vi "LV to ITX  Retrieve - HY TDMS.vi"(0 "File or Folder Path":path=path "C:/", 1 "Data Type":T2=enum."DAT", 2 "DAT header length":i32=11, 5 "offset":i32, 7 "length":i32=1, 9 "index":T3={"A"=1, "B"=0, "C"=2, "D"=0, "E"=3, "N1"=0, "N2"=0, "N3"=0, "N4"=0}, 11 "error in (no error)":errorcluster) -> (4 "A vs B":cluster{dbl[], dbl[]}[](graph), 6 "C vs D":cluster{dbl[], dbl[]}[](graph), 8 "E":dbl[][](graph), 10 "N":cluster{"N1":dbl, "N2":dbl, "N3":dbl, "N4":dbl}={"N1"=0.0624995231628418, "N2"=0.0624995231628418, "N3"=0.0624995231628418, "N4"=0.0624995231628418} {"N4" format="%#_6p"; "N3" format="%#_6p"; "N2" format="%#_6p"; "N1" format="%#_6p"}, 14 "Comments":string)   [LabVIEW 2016]
uses:
  <vilib>/Utility/miscctls.llb/LVOffsetAndMultiplierTypeDef.ctl
  <userlib>/LevyLab/LV to ITX/Typedefs/Retrieve Data Type.ctl
  <userlib>/LevyLab/LV to ITX/LVtoITX.lvclass
  <userlib>/LevyLab/Graph Utilities/graph_utilities.lvclass
panel:
  out "First element":dbl
  in  "X min & max":cluster{"Min":dbl, "Max":dbl}
  out "size(s)":i32[](array[numeric])
  out "last element":dbl
  in  "Manual input offset & multiplier for Ex ?":bool
  out "X Scale.Offset and Multiplier":T1
  in  "Specify data section ?":bool
  in  "Data length":i32=5000
  in  "Data offset":i32
  in  "D  is time?":bool
  in  "B is time?":bool
  out "time":string[][](table)
  in  "Use Folder Index File?":bool
  in  "Generate Folder Index File?":bool
  in  "Ez name":string="Ez name"
  in  "Ey name":string="Ey name"
  in  "Ex name":string="Ex name"
  in  "C y name":string="C y name"
  in  "D x name":string="D x name"
  in  "A y name":string="A y name"
  in  "B x name":string="B x name"
  out "Index, Wavenames":string[][](table)
  in  "recolor traces?":bool
  in  "Ex":T1={"Offset"=0.0, "Multiplier"=1.0}
  in  "Ey":T1={"Offset"=0.0, "Multiplier"=1.0}
  out "Path":path
  out "counter":i32
  out "pattern":string="*.dat"
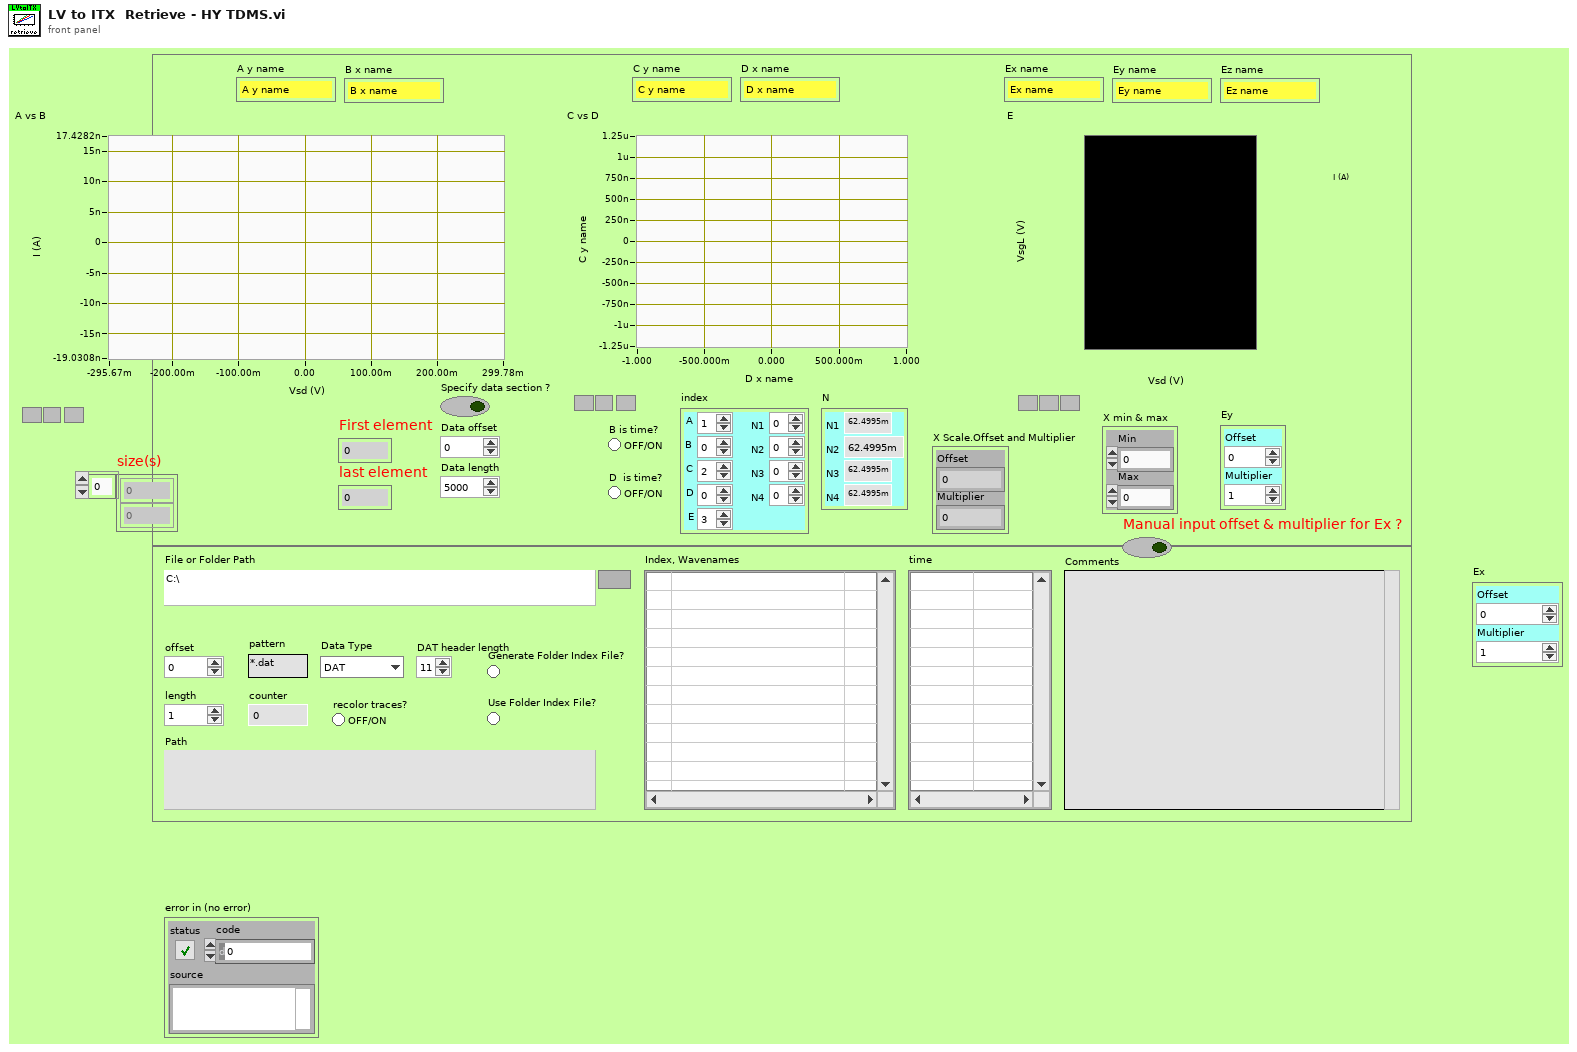
[diagram p1: front panel]
types:
  T1 = typedef "LVOffsetAndMultiplierTypeDef.ctl" = cluster{"Offset":dbl, "Multiplier":dbl}
  T2 = typedef "LVtoITX.lvclass/Retrieve Data Type.ctl" = enum16{"ITX", "ITX w/ 2D", "DAT", "TDMS"}
  T3 = cluster{"A":i32, "B":i32, "C":i32, "D":i32, "E":i32, "N1":i32, "N2":i32, "N3":i32, "N4":i32}
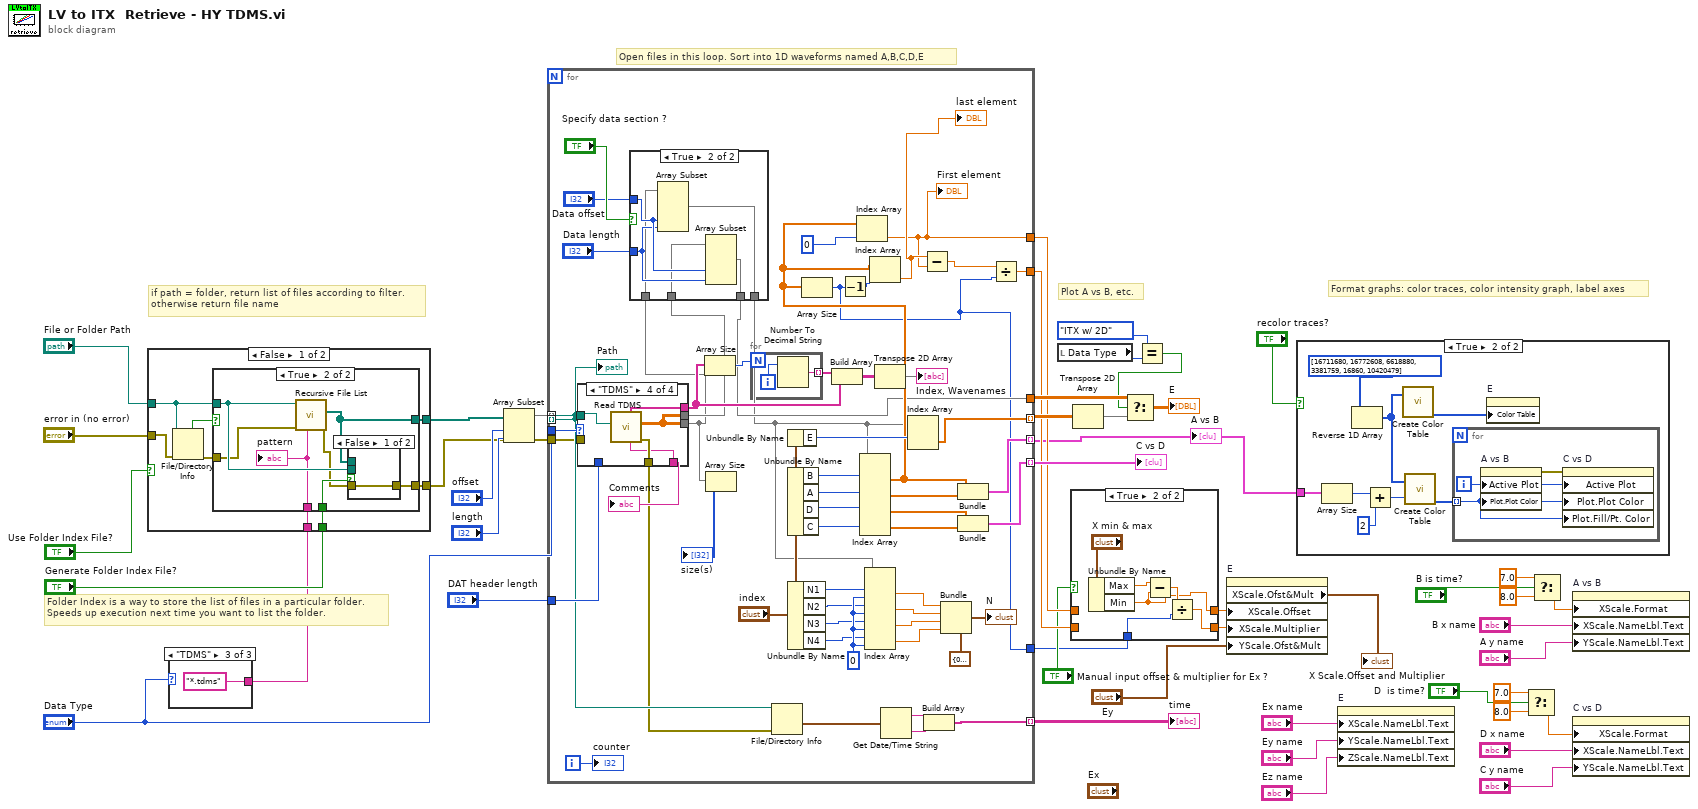
[diagram p0: block diagram]
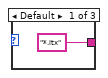
[diagram p3: hidden frame]
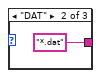
[diagram p4: hidden frame]
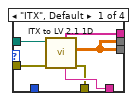
[diagram p7: hidden frame]
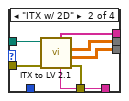
[diagram p8: hidden frame]
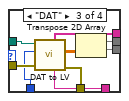
[diagram p9: hidden frame]
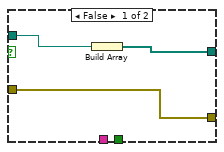
[diagram p10: hidden frame]
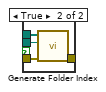
[diagram p11: hidden frame]
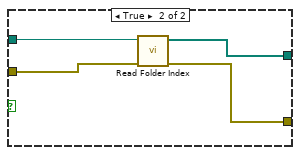
[diagram p12: hidden frame]
diagram:
  # "Plot A vs B, etc."
  # "Format graphs: color traces, color intensity graph, label axes"
  # "Open files in this loop. Sort into 1D waveforms named A,B,C,D,E"
  # "Folder Index is a way to store the list of files in a particular folder.\nSpeeds up execution next time you want to list the folder."
  # "if path = folder, return list of files according to filter.\notherwise return file name"
  n1 = case shown="\"TDMS\"" "Data Type" {
    tunnel: ["*.itx" ("pattern") "*.dat" ("pattern") "*.tdms" ("pattern")] -> w12
    frame Default {
    }
    frame "DAT" {
    }
    frame "TDMS" {
    }
  }
  n2 = case shown="False" "Use Folder Index File?" {
    tunnel: [w55 w75] -> w44
    tunnel: "File or Folder Path" -> [w57 w76]
    tunnel: "Generate Folder Index File?" -> [w54 _]
    tunnel: w12 -> [w53 _]
    tunnel: "error in (no error)" -> [w52 w74]
    tunnel: [w50 w73] -> w9
    frame False {
      n3 = File/Directory Info(path=w57, error in=w52) -> (directory=w56:bool, error out=w51:errorcluster)  [unwired: 5 out]
      n4 = case shown="True" w56 {
        tunnel: [w60 w66] -> w55
        tunnel: w57 -> [w59 w67]
        tunnel: w54 -> [_ w63]
        tunnel: w53 -> [_ w65]
        tunnel: w51 -> [w58 w64]
        tunnel: [w58 w61] -> w50
        frame False {
          n5 = Build Array(w59) -> (w60:path[])
        }
        frame True {
          n6 = call <vilib>:"Recursive File List.vi"("pattern"=w65, "error in (no error)"=w64, "Folder Path"=w67) -> ("error out"=w62:errorcluster, "All Files in Dir"=w66:path[])  [unwired: 4 in, 3 out]
          n7 = case shown="False" w63 {
            tunnel: w66 -> [_ w72]
            tunnel: w67 -> [_ w71]
            tunnel: w62 -> [w68 w70]
            tunnel: [w68 w69] -> w61
            frame False {
            }
            frame True {
              n8 = call <userlib>:"Generate Folder Index.vi"("error in (no error)"=w70, "File or Folder Path"=w71, "All Files in Dir"=w72) -> ("error out"=w69:errorcluster)  [unwired: 8 in]
            }
          }
          "pattern" <- w65
        }
      }
    }
    frame True {
      n9 = call <userlib>:"Read Folder Index.vi"("error in (no error)"=w74, "File or Folder Path"=w76) -> ("error out"=w73:errorcluster, "Files"=w75:path[])  [unwired: 8 in]
    }
  }
  n10 = Array Subset(array=w44, index="offset", length="length") -> (w25:path[])
  n11 = for {
    tunnel: w25 -> [w98] mode=indexing
    tunnel: [w98] -> _ mode=indexing
    tunnel: [w129] -> w2 mode=indexing
    tunnel: [w128] -> w35 mode=indexing
    tunnel: [w108] -> w39 mode=indexing
    tunnel: [w84] -> w37
    tunnel: [w102] -> w28 mode=indexing
    tunnel: "Data Type" -> [w100]
    tunnel: "DAT header length" -> [w99]
    tunnel: w9 -> [w97]
    tunnel: [w88] -> w5
    tunnel: [w77] -> w7
    tunnel: [w78] -> w1
    i -> [w131]
    w121 = 0 ("disabled index (col)")
    n12 = case shown="\"TDMS\"" w100 {
      tunnel: [w146 w153 w155 w163] -> w130
      tunnel: [w143 w150 w161 w166] -> w81
      tunnel: w98 -> [w147 w154 w162 w167]
      tunnel: [w142 w148 w156 w165] -> w122
      tunnel: [w143 w149 w161 w166] -> w85
      tunnel: w99 -> [_ _ w157 _]
      tunnel: w97 -> [w145 w151 w160 _]
      tunnel: [w144 w152 w159 w164] -> w96
      frame "ITX", Default {
        n13 = call <userlib>:"ITX to LV 2.1 1D.vi"("error in"=w145, "file (use dialog)"=w147) -> ("error out"=w144:errorcluster, "1D arrays"=w143:dbl[][], "Notes"=w146:string, "base wavenames"=w142:string[])  [unwired: 4 in, 2 out]
      }
      frame "ITX w/ 2D" {
        n14 = call <userlib>:"ITX to LV 2.1.vi"("error in"=w151, "file (use dialog)"=w154) -> ("error out"=w152:errorcluster, "1D arrays"=w150:dbl[][], "2D array"=w149:dbl[][], "Notes"=w153:string, "wave names"=w148:string[])  [unwired: 3 in, 2 out]
      }
      frame "DAT" {
        n15 = call <userlib>:"DAT to LV.vi"("error in (no error)"=w160, "header length"=w157, "File Path"=w162) -> ("error out"=w159:errorcluster, "Data"=w158:dbl[][], "Comments"=w155:string, "Wavenames"=w156:string[])  [unwired: 4 in, 1 out]
        n16 = Transpose 2D Array(2D array=w158) -> (transposed array=w161:dbl[][])
      }
      frame "TDMS" {
        n17 = call <userlib>:"Read TDMS.vi"("path"=w167) -> ("error out"=w164:errorcluster, "Data"=w166:dbl[][], "Comments"=w163:string, "Wavenames"=w165:string[])  [unwired: 4 in, 3 out]
      }
    }
    "Comments" <- w130
    n18 = case shown="True" "Specify data section ?" {
      tunnel: "Data offset" -> [_ w139]
      tunnel: "Data length" -> [_ w138]
      tunnel: w85 -> [w133 w137]
      tunnel: [w133 w136] -> w84
      tunnel: w81 -> [w132 w135]
      tunnel: [w132 w134] -> w83
      frame False {
      }
      frame True {
        n19 = Array Subset(array=w135, index (col)=w139, length (col)=w138) -> (w134:dbl[][])  [unwired: 2 in]
        n20 = Array Subset(array=w137, index (col)=w139, length (col)=w138) -> (w136:dbl[][])  [unwired: 2 in]
      }
    }
    n21 = Array Size(array=w122) -> (size(s)=w93:i32)
    n22 = Array Size(array=w81) -> (size(s)=→"size(s)":i32[])
    n23 = for {
      N: w93 -> [_]
      tunnel: [w140] -> w126 mode=indexing
      i -> [w141]
      n24 = Number To Decimal String(number=w141) -> (decimal integer string=w140:string)  [unwired: 1 in]
    }
    n25 = File/Directory Info(path=w98, error in=w96) -> (last mod=w101:timestamp)  [unwired: 6 out]
    n26 = Unbundle By Name("index") -> ("E"=w113:i32)
    n27 = Unbundle By Name("index") -> ("B"=w112:i32, "A"=w111:i32, "D"=w110:i32, "C"=w109:i32)
    n28 = Unbundle By Name("index") -> ("N1"=w114:i32, "N2"=w115:i32, "N3"=w116:i32, "N4"=w117:i32)
    n29 = Build Array(w126, w122) -> (w123:string[][])
    n30 = Index Array(array=w83, index (row) #1=w112, index (row) #2=w111, index (row) #3=w110, index (row) #4=w109) -> (element #1=w90:dbl[], element #2=w106:dbl[], element #3=w124:dbl[], element #4=w127:dbl[])  [unwired: 4 in]
    n31 = Array Size(array=w90) -> (size(s)=w78:i32)
    n32 = Decrement(x=w78) -> (x-1=w89:i32)
    n33 = Index Array(array=w90, index=0) -> (element=w77:dbl)
    "First element" <- w77
    n34 = Index Array(array=w83, index (row) #1=w114, index (col) #1=w121, index (row) #2=w115, index (col) #2=w121, index (row) #3=w116, index (col) #3=w121, index (row) #4=w117, index (col) #4=w121) -> (element #1=w103:dbl, element #2=w104:dbl, element #3=w105:dbl, element #4=w120:dbl)
    n35 = Index Array(array=w90, index=w89) -> (element=w79:dbl)
    "last element" <- w79
    n36 = Transpose 2D Array(2D array=w123) -> (transposed array=→"Index, Wavenames":string[][])
    n37 = Get Date/Time String(seconds (now)=w101) -> (date string=w94:string, time string=w95:string)  [unwired: 2 in]
    n38 = Index Array(array=w83, index (row)=w113) -> (element=w108:dbl[])  [unwired: 1 in]
    n39 = Subtract(x=w79, y=w77) -> (x-y=w82:dbl)
    n40 = Build Array(w94, w95) -> (w102:string[])
    n41 = Bundle(cluster=cluster{"N1":dbl, "N2":dbl, "N3":dbl, "N4":dbl} {"N1"=0.0, "N2"=0.0, "N3"=0.0, "N4"=0.0}, "N1"=w103, "N2"=w104, "N3"=w105, "N4"=w120) -> (→"N":cluster{"N1":dbl, "N2":dbl, "N3":dbl, "N4":dbl})
    n42 = Bundle("Data"=w90, "Data"=w106) -> (w129:cluster{"Data":dbl[], "Data":dbl[]})  [unwired: 1 in]
    n43 = Bundle("Data"=w124, "Data"=w127) -> (w128:cluster{"Data":dbl[], "Data":dbl[]})  [unwired: 1 in]
    n44 = Divide(x=w82, y=w78) -> (x/y=w88:dbl)
    "counter" <- w131
    "Path" <- w98
  }
  "A vs B" <- w2
  "C vs D" <- w35
  "time" <- w28
  n45 = local read "Data Type"() -> (w15:T2)
  n46 = case shown="True" "Manual input offset & multiplier for Ex ?" {
    tunnel: w7 -> [w169 _]
    tunnel: [w169 w170] -> w6
    tunnel: w5 -> [w168 _]
    tunnel: [w168 w171] -> w4
    tunnel: w1 -> [_ w173]
    frame False {
    }
    frame True {
      n47 = Unbundle By Name("X min & max") -> ("Max"=w174:dbl, "Min"=w170:dbl)
      n48 = Subtract(x=w174, y=w170) -> (x-y=w172:dbl)
      n49 = Divide(x=w172, y=w173) -> (x/y=w171:dbl)
    }
  }
  n50 = Transpose 2D Array(2D array=w39) -> (transposed array=w40:dbl[][])
  n51 = Equal?(x=enum16{"ITX", "ITX w/ 2D", "DAT"}."ITX w/ 2D" ("Enum"), y=w15) -> (x = y?=w13:bool)
  n52 = Select(t=w37, s=w13, f=w40) -> (s? t:f=→"E":dbl[][])
  n53 = property on="E" class="IntGraph (strict)"("XScale.Offset"=w6, "XScale.Multiplier"=w4, "YScale.Ofst&Mult"="Ey") -> ("XScale.Ofst&Mult"=→"X Scale.Offset and Multiplier":T1)  [unwired: 2 in, 2 out]
  n54 = case shown="True" "recolor traces?" {
    tunnel: w2 -> [_ w178]
    frame False {
    }
    frame True {
      n55 = Array Size(array=w178) -> (size(s)=w179:i32)
      n56 = Reverse 1D Array(array=u32[] [16711680, 16772608, 6618880, 3381759, 16860, 10420479] ("color scale")) -> (reversed array=w177:u32[])
      n57 = Add(x=w179, y=2 ("x")) -> (x+y=w183:i32)
      n58 = call <userlib>:"Create Color Table.vi"("Colors []"=w177) -> ("Color Tbl"=w181:u32[])  [unwired: 1 in, 3 out]
      n59 = call <userlib>:"Create Color Table.vi"("Colors []"=w177, "Size (256)"=w183) -> ("Color Tbl"=w180:u32[])  [unwired: 3 out]
      n60 = for {
        tunnel: w180 -> [w184] mode=indexing
        i -> [w185]
        n61 = property on="A vs B" class="XYGraph (strict)"("Active Plot"=w185, "Plot.Plot Color"=w184) -> (error out=w186:errorcluster)  [unwired: 2 in, 1 out]
        n62 = property on="C vs D" class="XYGraph (strict)"(error in=w186, "Active Plot"=w185, "Plot.Plot Color"=w184, "Plot.Fill/Pt. Color"=w184) -> ()  [unwired: 1 in, 2 out]
      }
      n63 = property on="E" class="IntGraph (strict)"("Color Table"=w181) -> ()  [unwired: 2 in, 2 out]
    }
  }
  n64 = property on="E" class="IntGraph (strict)"("XScale.NameLbl.Text"="Ex name", "YScale.NameLbl.Text"="Ey name", "ZScale.NameLbl.Text"="Ez name") -> ()  [unwired: 2 in, 2 out]
  n65 = Select(t=7.0, s="D  is time?", f=8.0) -> (s? t:f=w21:dbl)
  n66 = Select(t=7.0, s="B is time?", f=8.0) -> (s? t:f=w22:dbl)
  n67 = property on="A vs B" class="XYGraph (strict)"("XScale.Format"=w22, "XScale.NameLbl.Text"="B x name", "YScale.NameLbl.Text"="A y name") -> ()  [unwired: 2 in, 2 out]
  n68 = property on="C vs D" class="XYGraph (strict)"("XScale.Format"=w21, "XScale.NameLbl.Text"="D x name", "YScale.NameLbl.Text"="C y name") -> ()  [unwired: 2 in, 2 out]
